vi "r_dot_growth.vi"(10 "Sat pol in":dbl, 11 "r array in":dbl[](array[numeric])) -> (3 "r dot out":dbl[](array[numeric]))   [LabVIEW 2018]
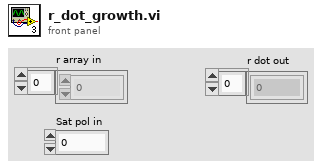
[diagram p1: front panel]
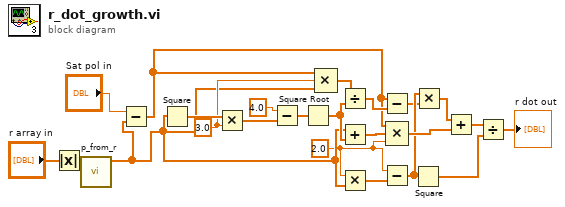
[diagram p0: block diagram]
diagram:
  w3 = 2.0
  w7 = 3.0
  n1 = Absolute Value(x="r array in") -> (abs(x)=w1:dbl[])
  n2 = call "p_from_r.vi"("r array in"=w1) -> ("P eff. out"=w6:dbl[])  [unwired: 10 in]
  n3 = Subtract(x="Sat pol in", y=w6) -> (x-y=w2:dbl[])
  n4 = Square(x=w6) -> (x^2=w22:dbl[])
  n5 = Multiply(x=w22, y=w7) -> (x*y=w14:dbl[])
  n6 = Subtract(x=4.0, y=w14) -> (x-y=w20:dbl[])
  n7 = Square Root(x=w20) -> (sqrt(x)=w10:dbl[])
  n8 = Compound Arithmetic op=MULTIPLY(w2, w7, w6) -> (w5:dbl[])
  n9 = Divide(x=w5, y=w10) -> (x/y=w4:dbl[])
  n10 = Add(x=w6, y=w10) -> (x+y=w11:dbl[])
  n11 = Multiply(x=w3, y=w6) -> (x*y=w12:dbl[])
  n12 = Subtract(x=w2, y=w4) -> (x-y=w13:dbl[])
  n13 = Subtract(x=w3, y=w12) -> (x-y=w15:dbl[])
  n14 = Compound Arithmetic op=MULTIPLY(w2, w11, w3) -> (w19:dbl[])
  n15 = Square(x=w15) -> (x^2=w16:dbl[])
  n16 = Multiply(x=w15, y=w13) -> (x*y=w18:dbl[])
  n17 = Add(x=w18, y=w19) -> (x+y=w17:dbl[])
  n18 = Divide(x=w17, y=w16) -> (x/y=→"r dot out":dbl[])
